vi "缓冲区数据曲线生成.vi"(8 "错误输入（无错误）":errorcluster, 9 "坐标轴映射":T1, 10 "曲线设置":T2={"X轴数据选择"=enum."设置电压", "Y轴组"=[]}, 11 "数据缓冲输入":refnum<queue>) -> (0 "错误输出":errorcluster, 2 "曲线":cluster{dbl[], dbl[]}[](array[cluster]), 3 "数据缓冲输出":refnum<queue>)   [LabVIEW 2020]
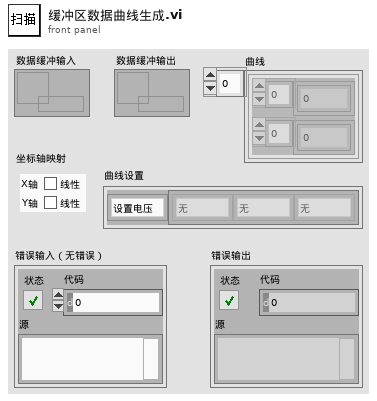
[diagram p1: front panel]
types:
  T1 = typedef "坐标轴映射.ctl" = cluster{"X轴":bool, "Y轴":bool}
  T2 = typedef "曲线设置.ctl" = cluster{"X轴数据选择":enum16{"时间", "设置电压", "读取电流", "读取电压"}, "Y轴组":enum16{"时间", "设置电压", "读取电流", "读取电压", "无"}[]}
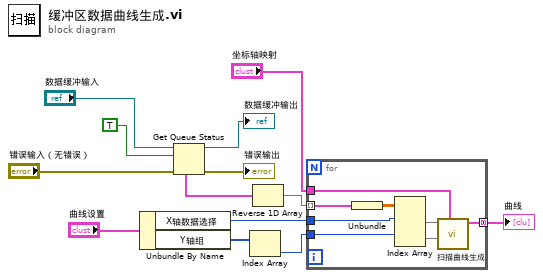
[diagram p0: block diagram]
diagram:
  n1 = Unbundle By Name("曲线设置") -> ("X轴数据选择"=w12:enum16{"时间", "设置电压", "读取电流", "读取电压"}, "Y轴组"=w11:enum16{"时间", "设置电压", "读取电流", "读取电压", "无"}[])
  n2 = Get Queue Status(queue="数据缓冲输入", return elements? (F)=TRUE ("返回元素？(F)"), error in (no error)="错误输入（无错误）") -> (queue out=→"数据缓冲输出":refnum<queue>, error out=→"错误输出":errorcluster, elements=w6:cluster{"测试数据":dbl[][]}[])  [unwired: 5 out]
  n3 = Index Array(array=w11) -> (element=w13:enum16{"时间", "设置电压", "读取电流", "读取电压", "无"})  [unwired: 1 in]
  n4 = Reverse 1D Array(array=w6) -> (reversed array=w2:cluster{"测试数据":dbl[][]}[])
  n5 = for {
    tunnel: w13 -> [w21]
    tunnel: w12 -> [w20]
    tunnel: [w17] -> w1 mode=concatenating
    tunnel: "坐标轴映射" -> [w16]
    tunnel: w2 -> [w15] mode=indexing
    n6 = Unbundle(w15) -> ("测试数据"=w14:dbl[][])
    n7 = Index Array(array=w14, index (row) #1=w20, index (row) #2=w21) -> (element #1=w18:dbl[], element #2=w19:dbl[])  [unwired: 2 in]
    n8 = call "扫描曲线生成.vi"("坐标轴映射"=w16, "Y"=w19, "X"=w18) -> ("曲线"=w17:cluster{dbl[], dbl[]}[])  [unwired: 7 in, 1 out]
  }
  "曲线" <- w1
